vi "checkFreq.vi"(1 "Path":path, 4 "error in":errorcluster, 5 "Set Frequency":dbl, 6 "Wave generator":string, 7 "Lock-In":string) -> (0 "error out":errorcluster, 2 "Amplitude":dbl, 3 "Phase Shift":dbl)   [LabVIEW 2010]
uses:
  <vilib>/Utility/file.llb/Write To Spreadsheet File (DBL).vi
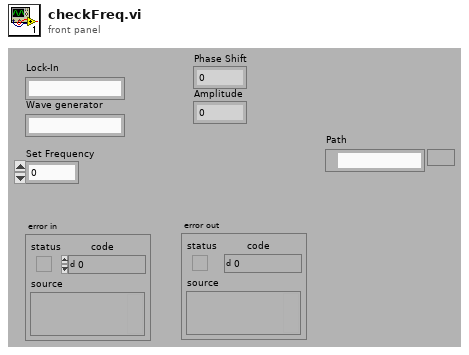
[diagram p1: front panel]
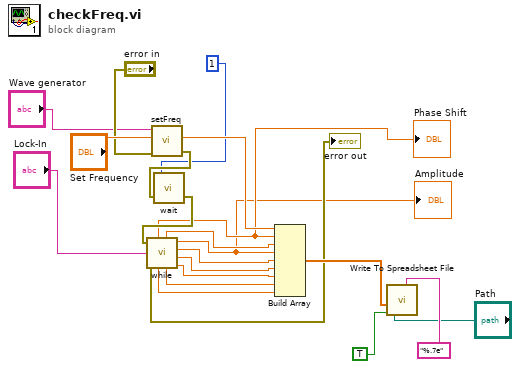
[diagram p0: block diagram]
diagram:
  n1 = call "setFreq.vi"("error in"="error in", "Frequenz in Hz"="Set Frequency", "address string"="Wave generator") -> ("error out"=w11:errorcluster)  [unwired: 3 in]
  n2 = call "wait.vi"("error in"=w11, "Wartezeit in Sek"=1) -> ("error out"=w10:errorcluster)  [unwired: 1 in]
  n3 = call "while.vi"("error in"=w10, "adress string"="Lock-In") -> ("Phase Shift"=w2:dbl, "error out"=→"error out":errorcluster, "Errror U2"=w8:dbl, "Error PS"=w3:dbl, "Amplitude"=w1:dbl, "Error  Amp"=w4:dbl, "U2"=w7:dbl, "U1"=w5:dbl, "Error U1"=w6:dbl)
  "Phase Shift" <- w2
  "Amplitude" <- w1
  n4 = Build Array("Set Frequency", w2, w3, w1, w4, w5, w6, w7, w8) -> (w17:dbl[])
  n5 = call-poly <vilib>:"Write To Spreadsheet File.vi"("format (%.3f)"="%.7e", "append to file? (new file:F)"=TRUE, "1D data"=w17, "file path (dialog if empty)"="Path") -> ()  [unwired: 4 in, 1 out]
